vi "Get Strings from Ref.vi"(8 "error in (no error)":errorcluster, 9 "Label Prefix":string, 10 "GObj Refnum in":refnum<vi>, 11 "WaveformGraph in":refnum<class "WaveformGraph.lvclass">) -> (0 "error out":errorcluster, 1 "Valid?":bool, 2 "GObj Refnum out":refnum<vi>, 3 "WaveformGraph out":refnum<class "WaveformGraph.lvclass">, 4 "GObj Name":string)   [LabVIEW 2013, in "SET Project Data.lvlib" / "WaveformGraph.lvclass"]
uses:
  WaveformGraph.lvclass
  GraphChart/GraphChart.lvclass
  GObject/GObject.lvclass/GObject.ctl
  GObject/Write UID.vi
  SET Project Data.lvlib
  GObject/GObject.lvclass
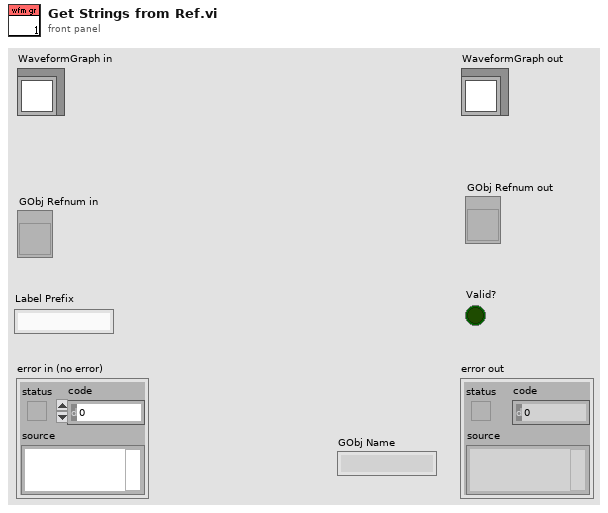
[diagram p1: front panel]
types:
  T1 = typedef "LVCursorListTypeDef.ctl" = cluster{"Name":string, "Color":u32, "Style":u8, "Point Style":u8, "Name Visible":bool, "Allow Drag":bool, "Cursor Mode":u32, "Plot":i32, "Index":i32, "Position":cluster{"X":dbl, "Y":dbl}, "X Scale":u32, "Y Scale":u32, "Watch Plots":i32[], "Watch All Plots":bool, "Plot Area":i32, "Label Offset":cluster{"X":dbl, "Y":dbl}}[]
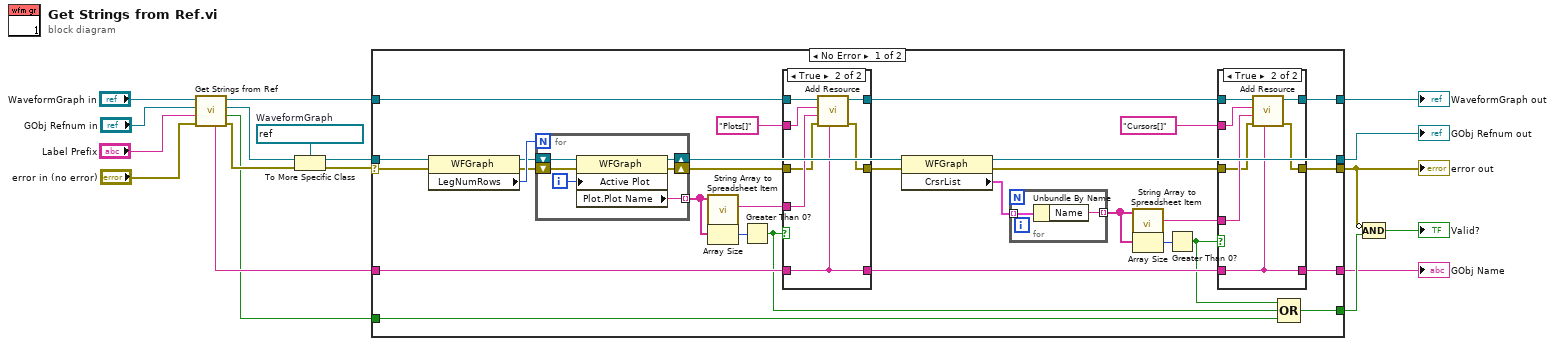
[diagram p0: block diagram]
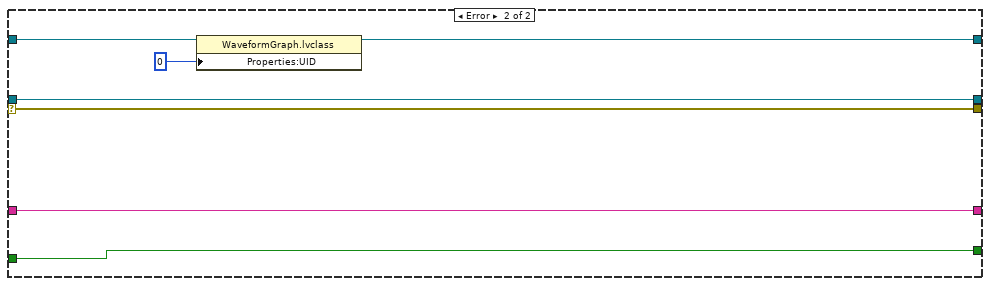
[diagram p4: hidden frame]
diagram:
  w13 = refnum<vi> refnum  # WaveformGraph
  n1 = call-parent "Get Strings from Ref.vi"("error in (no error)"="error in (no error)", "Label Prefix"="Label Prefix", "GObj Refnum in"="GObj Refnum in", "GraphChart in"="WaveformGraph in") -> ("error out"=w9:errorcluster, "Valid?"=w7:bool, "GObj Refnum out"=w10:refnum<vi>, "GraphChart out"=w11:refnum<class "WaveformGraph.lvclass">, "GObj Name"=w8:string)  [unwired: 3 in]
  n2 = To More Specific Class(target class=w13, reference=w10, error in=w9) -> (specific class reference=w6:refnum<vi>, error out=w12:errorcluster)
  n3 = case shown="No Error" w12 {
    selector: w12 -> [w35 w82]
    tunnel: w6 -> [w36 w83]
    tunnel: w11 -> [w46 w81]
    tunnel: [w26 w79] -> w5
    tunnel: [w19 w82] -> w2
    tunnel: [w28 w83] -> w4
    tunnel: w8 -> [w43 w78]
    tunnel: w7 -> [w41 w77]
    tunnel: [w22 w78] -> w1
    tunnel: [w40 w77] -> w14
    frame No Error {
      n4 = property class="WFGraph"(reference=w36, error in=w35) -> (reference out=w38:refnum<vi>, error out=w37:errorcluster, "LegNumRows"=w39:u32)
      n5 = for {
        N: w39 -> [_]
        shift-right: [w65] -> w32
        shift-left: w38 -> [w66]
        shift-right: [w62] -> w34
        shift-left: w37 -> [w63]
        tunnel: [w61] -> w33 mode=indexing
        i -> [w64]
        n6 = property class="WFGraph"(reference=w66, error in=w63, "Active Plot"=w64) -> (reference out=w65:refnum<vi>, error out=w62:errorcluster, "Plot.Plot Name"=w61:string)
      }
      n7 = call "String Array to Spreadsheet Item.vi"("Strings [] (ASCII)"=w33) -> ("Spreadsheet Item (ASCII)"=w44:string)  [unwired: 10 in]
      n8 = Array Size(array=w33) -> (size(s)=w48:i32)
      n9 = Greater Than 0?(x=w48) -> (x > 0?=w42:bool)
      n10 = case shown="True" w42 {
        tunnel: w46 -> [w69 w76]
        tunnel: [w69 w75] -> w27
        tunnel: w43 -> [w68 w72]
        tunnel: w44 -> [_ w74]
        tunnel: "Plots[]" -> [_ w73]
        tunnel: [w68 w72] -> w23
        tunnel: w34 -> [w67 w71]
        tunnel: [w67 w70] -> w31
        frame False {
        }
        frame True {
          n11 = call "Add Resource.vi"("TagPrefix"=w72, "error in (no error)"=w71, "ItemText"=w74, "ItemName"=w73, "GObject in"=w76) -> ("error out"=w70:errorcluster, "GObject out"=w75:refnum<class "WaveformGraph.lvclass">)  [unwired: 5 in]
        }
      }
      n12 = property class="WFGraph"(reference=w32, error in=w31) -> (reference out=w28:refnum<vi>, error out=w29:errorcluster, "CrsrList"=w30:T1)
      n13 = for {
        tunnel: w30 -> [w60] mode=indexing
        tunnel: [w59] -> w21 mode=indexing
        n14 = Unbundle By Name(w60) -> ("Name"=w59:string)
      }
      n15 = call "String Array to Spreadsheet Item.vi"("Strings [] (ASCII)"=w21) -> ("Spreadsheet Item (ASCII)"=w24:string)  [unwired: 10 in]
      n16 = Array Size(array=w21) -> (size(s)=w47:i32)
      n17 = Greater Than 0?(x=w47) -> (x > 0?=w20:bool)
      n18 = case shown="True" w20 {
        tunnel: w27 -> [w51 w58]
        tunnel: [w51 w57] -> w26
        tunnel: w23 -> [w50 w54]
        tunnel: w24 -> [_ w56]
        tunnel: "Cursors[]" -> [_ w55]
        tunnel: [w50 w54] -> w22
        tunnel: w29 -> [w49 w53]
        tunnel: [w49 w52] -> w19
        frame False {
        }
        frame True {
          n19 = call "Add Resource.vi"("TagPrefix"=w54, "error in (no error)"=w53, "ItemText"=w56, "ItemName"=w55, "GObject in"=w58) -> ("error out"=w52:errorcluster, "GObject out"=w57:refnum<class "WaveformGraph.lvclass">)  [unwired: 5 in]
        }
      }
      n20 = Compound Arithmetic op=OR(w20, w42, w41) -> (w40:bool)
    }
    frame Error {
      n21 = property class="WaveformGraph.lvclass"(reference=w81, "Properties:UID"=0 ("UID")) -> (reference out=w79:refnum<class "WaveformGraph.lvclass">)  [unwired: 1 in, 1 out]
    }
  }
  "error out" <- w2
  "WaveformGraph out" <- w5
  "GObj Refnum out" <- w4
  "GObj Name" <- w1
  n22 = Compound Arithmetic op=AND(invert w2, w14) -> (→"Valid?":bool)
